vi "Convert From Base64 and Store.vi"(8 "error in (no error)":errorcluster, 9 "File Path":path, 11 "Base64 String":string) -> (0 "error out":errorcluster, 3 "String":string)   [LabVIEW 2014, in "FrontPanelPublisher.lvlib"]
uses:
  FrontPanelPublisher.lvlib
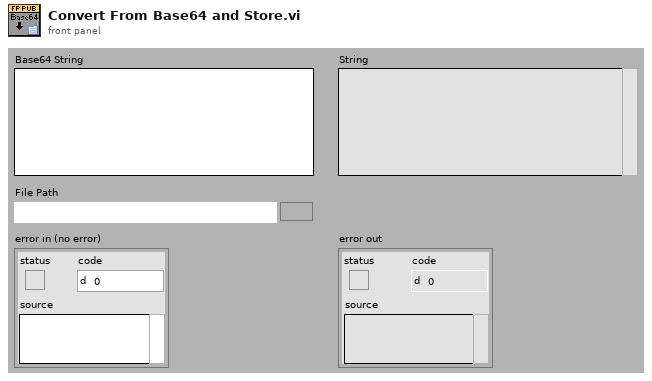
[diagram p1: front panel]
types:
  T1 = enum16{"open", "replace", "create", "open or create", "replace or create", "replace or create with confirmation"}
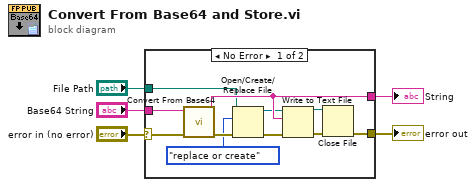
[diagram p0: block diagram]
diagram:
  n1 = case shown="No Error" "error in (no error)" {
    selector: "error in (no error)" -> [w14 w17]
    tunnel: [w16 w17] -> w5
    tunnel: "Base64 String" -> [w15 _]
    tunnel: [w12 _] -> w2
    tunnel: "File Path" -> [w6 _]
    frame No Error {
      n2 = call "Convert From Base64.vi"("error in (no error)"=w14, "Base64 String"=w15) -> ("error out"=w13:errorcluster, "String"=w12:string)  [unwired: 8 in]
      n3 = Open/Create/Replace File(file path (use dialog)=w6, error in=w13, operation (0:open)=T1."replace or create") -> (refnum out=w8:refnum<file>, error out=w11:errorcluster)  [unwired: 4 out]
      n4 = Write to Text File(file (use dialog)=w8, text=w12, error in=w11) -> (refnum out=w9:refnum<file>, error out=w10:errorcluster)  [unwired: 1 in, 1 out]
      n5 = Close File(refnum=w9, error in=w10) -> (error out=w16:errorcluster)  [unwired: 1 out]
    }
    frame Error {
    }
  }
  "String" <- w2
  "error out" <- w5
